vi "AR-DI-create.vi"(8 "error in":errorcluster, 11 "lines":tag="Dev1/port1/line0:2") -> (0 "error out":errorcluster, 3 "DI task out":refnum<k21>)   [LabVIEW 2021]
uses:
  <vilib>/DAQmx/create/channels.llb/DAQmx Create Channel (DI-Digital Input).vi
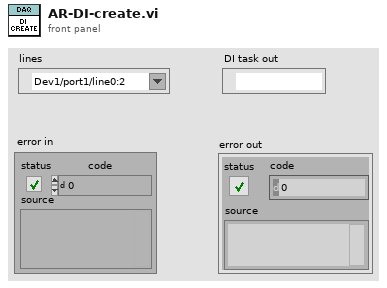
[diagram p1: front panel]
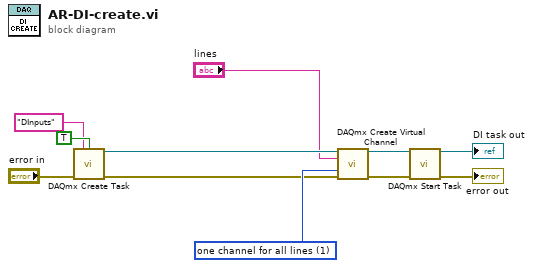
[diagram p0: block diagram]
diagram:
  w6 = 1 items=["one channel for each line", "one channel for all lines"] ("line grouping")
  n1 = call <vilib>:"DAQmx Create Task.vi"("new task name"="DInputs", "auto cleanup"=TRUE, "error in"="error in") -> ("task out"=w8:refnum<k21>, "error out"=w1:errorcluster)  [unwired: 11 in]
  n2 = call-poly <vilib>:"DAQmx Create Virtual Channel.vi"("task in"=w8, "lines"="lines", "line grouping"=w6, "error in"=w1) -> ("task out"=w7:refnum<k21>, "error out"=w9:errorcluster)  [unwired: 10 in]
  n3 = call <vilib>:"DAQmx Start Task.vi"("task/channels in"=w7, "error in"=w9) -> ("task out"=→"DI task out":refnum<k21>, "error out"=→"error out":errorcluster)  [unwired: 12 in]
